vi "6（发送方）.vi"() -> ()   [LabVIEW 2017]
uses:
  <vilib>/Analysis/NI_AALBase.lvlib
panel:
  out "波形图表":dbl[](graph)
  in  "停止":bool
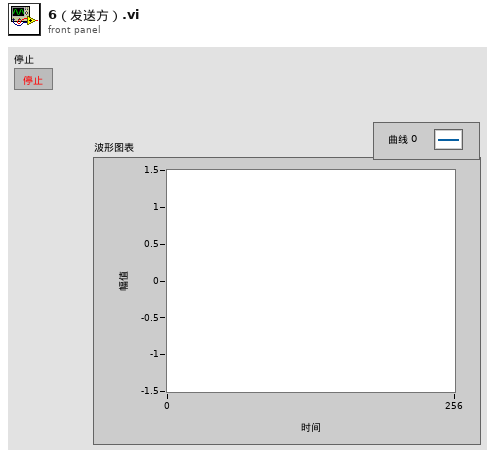
[diagram p1: front panel]
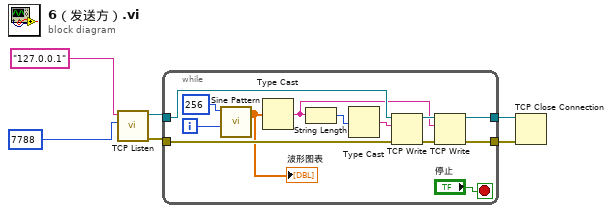
[diagram p0: block diagram]
diagram:
  n1 = call <vilib>:"TCP Listen.vi"("port"=u16 7788 ("远程端口或服务名称"), "service name"="127.0.0.1" ("地址")) -> ("error out"=w3:errorcluster, "connection ID"=w4:refnum<k5>)  [unwired: 5 in, 3 out]
  n2 = while {
    tunnel: w4 -> [w17]
    tunnel: w3 -> [w16]
    tunnel: [w9] -> w6
    tunnel: [w8] -> w5
    i -> [w19]
    stop <- "停止" stop-if-true
    n3 = call <vilib>:"Sine Pattern.vi"("phase(degrees)"=w19, "samples"=256) -> ("Sinusoidal Pattern"=w7:dbl[])  [unwired: 2 in, 1 out]
    "波形图表" <- w7
    n4 = Type Cast(x=w7) -> (*(type *) &x=w10:string)  [unwired: 1 in]
    n5 = String Length(string=w10) -> (length=w12:i32)
    n6 = Type Cast(x=w12) -> (*(type *) &x=w11:string)  [unwired: 1 in]
    n7 = TCP Write(connection ID=w17, data in=w11, error in (no error)=w16) -> (connection ID out=w14:refnum<k5>, error out=w13:errorcluster)  [unwired: 1 in, 1 out]
    n8 = TCP Write(connection ID=w14, data in=w10, error in (no error)=w13) -> (connection ID out=w9:refnum<k5>, error out=w8:errorcluster)  [unwired: 1 in, 1 out]
  }
  n9 = TCP Close Connection(connection ID=w6, error in (no error)=w5) -> ()  [unwired: 1 in, 2 out]
